vi "Workspace Tool Test.vi"() -> ()   [LabVIEW 2016]
uses:
  <vilib>/NI Veristand/Execution/Project/NI VeriStand - Send Workspace Tool Message (String).vi
  <vilib>/NI Veristand/Execution/Project/NI_VS Project ExecutionAPI.lvlib
panel:
  in  "Send Event":bool
  in  "Data":string="Merda1"
  in  "Command":string="My Command"
  in  "Stop":bool
  in  "Project File Path":path=path "C:/Users/Public/Documents/National Instruments/NI VeriStand 2013/Projects/Example/Sinewave Delay.nivsproj"
  in  "Workspace Tool Path":path=path "C:/Program Files (x86)/National Instruments/VeriStand 2013/NI VeriStand.exe/NI VeriStand/Workspace/Tools/scr_TDMS Data Viewer.vi"
  out "response":string="Reply"
  # "Tools to be tested ->"
  # "C:\\Users\\Public\\Documents\\National Instruments\\NI VeriStand 2013\\Projects\\Multi_WS\\Custom Tool\\MyLLB.llb\\FM_WS_tool.vi"
  # "C:\\Program Files (x86)\\National Instruments\\VeriStand 2013\\NI VeriStand.exe\\NI VeriStand\\Workspace\\Tools\\scr_TDMS Data Viewer.vi"
  # "USE RELATIVE PATHS for built-in tools"
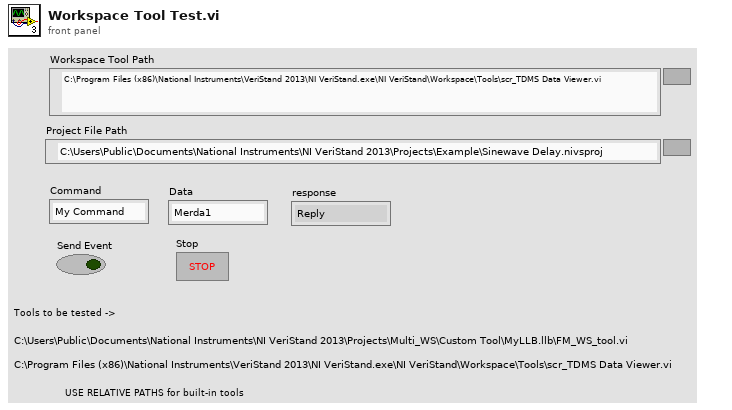
[diagram p1: front panel]
types:
  T1 = typedef "NI_VS Project ExecutionAPI.lvlib/Project Ref.ctl" = refnum<k24>
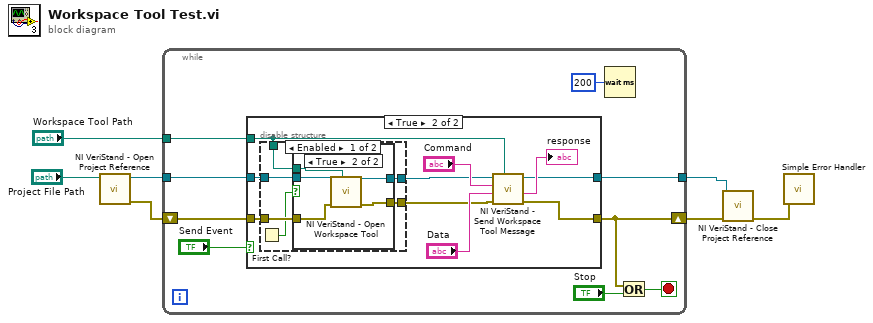
[diagram p0: block diagram]
diagram:
  n1 = call <vilib>:"NI VeriStand - Open Project Reference.vi"("Project File Path"="Project File Path") -> ("error out"=w7:errorcluster, "Project Ref"=w6:T1)  [unwired: 9 in]
  n2 = while {
    tunnel: w6 -> [w15]
    tunnel: "Workspace Tool Path" -> [w14]
    shift-right: [w11] -> w3
    shift-left: w7 -> [w16]
    tunnel: [w8] -> w1
    stop <- w13 stop-if-true
    n3 = case shown="True" "Send Event" {
      tunnel: w16 -> [w18 w22]
      tunnel: w15 -> [w17 w23]
      tunnel: w14 -> [_ w19]
      tunnel: [w18 w25] -> w11
      tunnel: [w17 w24] -> w8
      frame False {
      }
      frame True {
        n4 = disable-structure shown="Enabled" {
          disable-tunnel: w23 -> [w34 w43]
          disable-tunnel: w22 -> [w33 w42]
          disable-tunnel: [w32 w43] -> w21
          disable-tunnel: [w30 w42] -> w20
          disable-tunnel: w19 -> [w29 _]
          frame Enabled {
            n5 = First Call?() -> (First Call?: T/F=w31:bool)
            n6 = case shown="True" w31 {
              tunnel: w34 -> [w36 w41]
              tunnel: w33 -> [w35 w39]
              tunnel: [w36 w40] -> w32
              tunnel: [w35 w38] -> w30
              tunnel: w29 -> [_ w37]
              frame False {
              }
              frame True {
                n7 = call <vilib>:"NI VeriStand - Open Workspace Tool.vi"("Workspace Tool Path"=w37, "error in (no error)"=w39, "Project Ref in"=w41) -> ("error out"=w38:errorcluster, "Project Ref out"=w40:T1)  [unwired: 7 in]
              }
            }
          }
          frame Disabled {
          }
        }
        n8 = call-poly <vilib>:"NI VeriStand - Send Workspace Tool Message.vi"("Workspace Tool Path"=w19, "error in (no error)"=w20, "Data"="Data", "Command"="Command", "Project Ref in"=w21) -> ("error out"=w25:errorcluster, "response"=→"response":string, "Project Ref out"=w24:T1)  [unwired: 4 in]
      }
    }
    n9 = Wait (ms)(milliseconds to wait=u32 200) -> ()  [unwired: 1 out]
    n10 = Or(x=w11, y="Stop") -> (x .or. y?=w13:bool)
  }
  n11 = call <vilib>:"NI VeriStand - Close Project Reference.vi"("error in (no error)"=w3, "Project Ref"=w1) -> ("error out"=w2:errorcluster)  [unwired: 9 in]
  n12 = call <vilib>:"Simple Error Handler.vi"("error in (no error)"=w2) -> ()  [unwired: 4 in, 5 out]
